vi "Prasing Frame.vi"(8 "error in (no error)":errorcluster caption="entrée d'erreur (pas d'erreur)", 11 "Class UART Enocean en entrée":refnum<class "Class UART Enocean.lvclass">) -> (0 "error out":errorcluster caption="sortie d'erreur", 3 "Class UART Enocean en sortie":refnum<class "Class UART Enocean.lvclass">)   [LabVIEW 2020, in "Library Instrument & Equipement.lvlib" / "Library UART.lvlib" / "Class UART Enocean.lvclass"]
uses:
  Class UART Enocean.lvclass
  C:/Users/ngarcin/OneDrive - Altyor/Standard TB/Class/UART/UART (Default)/Class UART (Default).lvclass
  Class UART Enocean.lvclass/Class UART Enocean.ctl
  Commun VI/Library Commun.lvlib
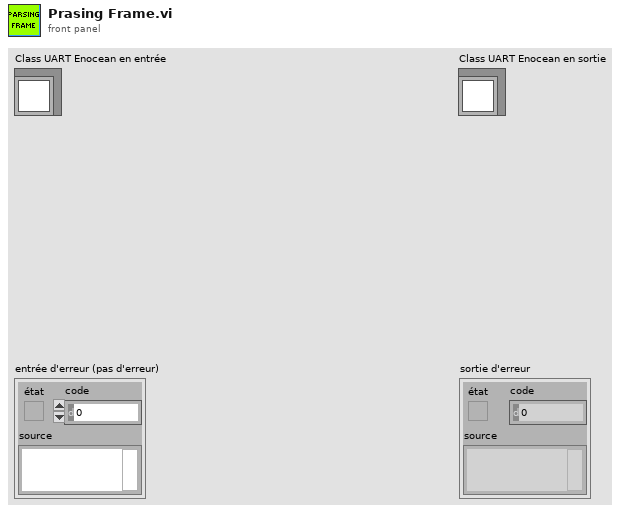
[diagram p1: front panel]
types:
  T1 = enum16{"Wait Synchro bit", "Wait Size Header", "Check CRC Header", "Wait Size Data", "Wait Size Optional", "Check CRC Data", "Extract Data"}[]
  T2 = enum16{"CRC Altyor", "CRC Xor On all Bytes", "CRC8", "CRC16", "CRC32", "Other"}
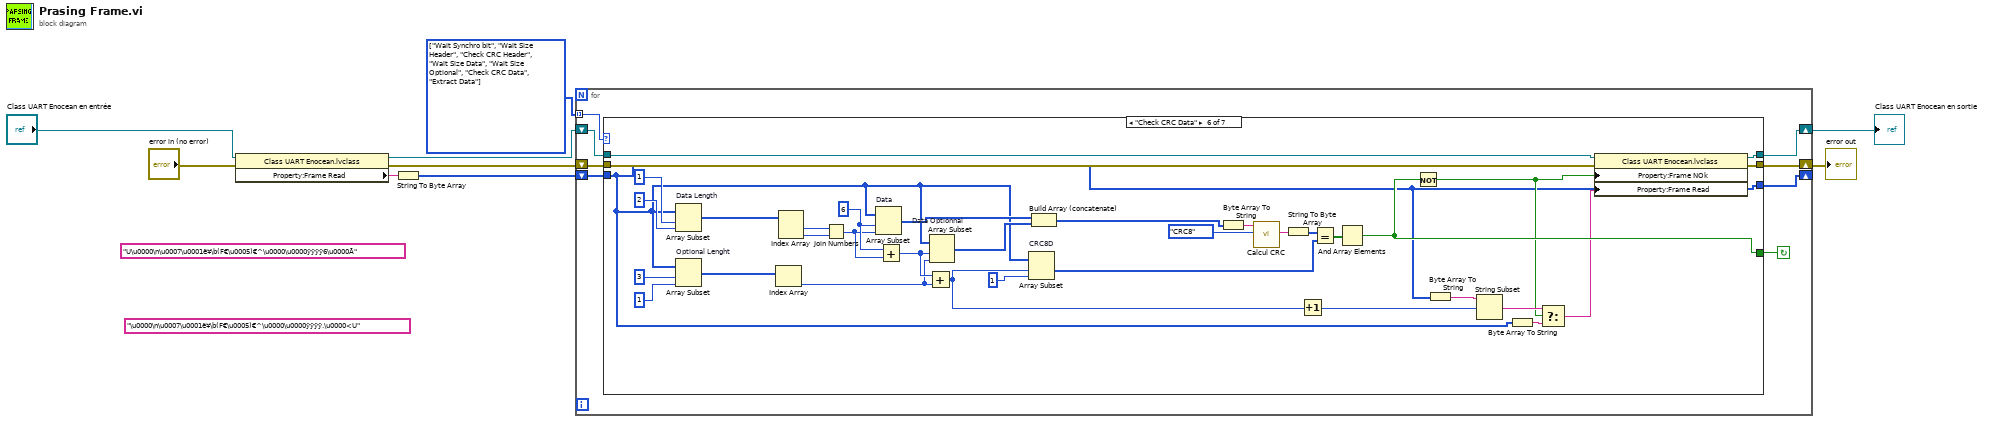
[diagram p0: block diagram]
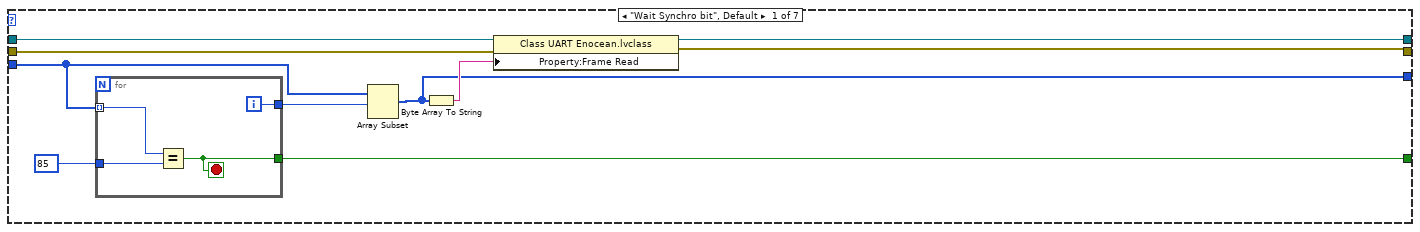
[diagram p2: hidden frame]
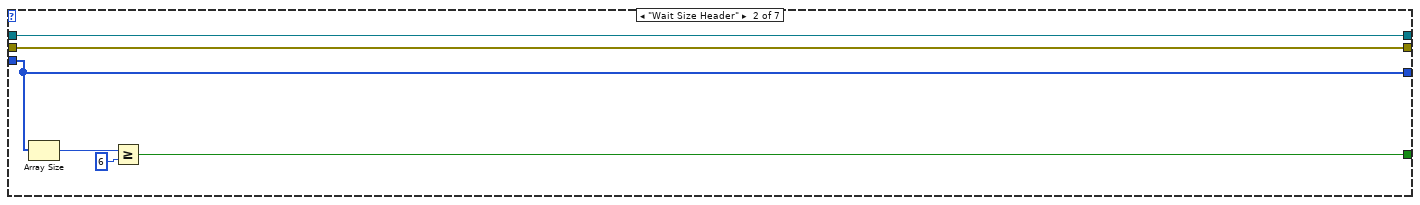
[diagram p3: hidden frame]
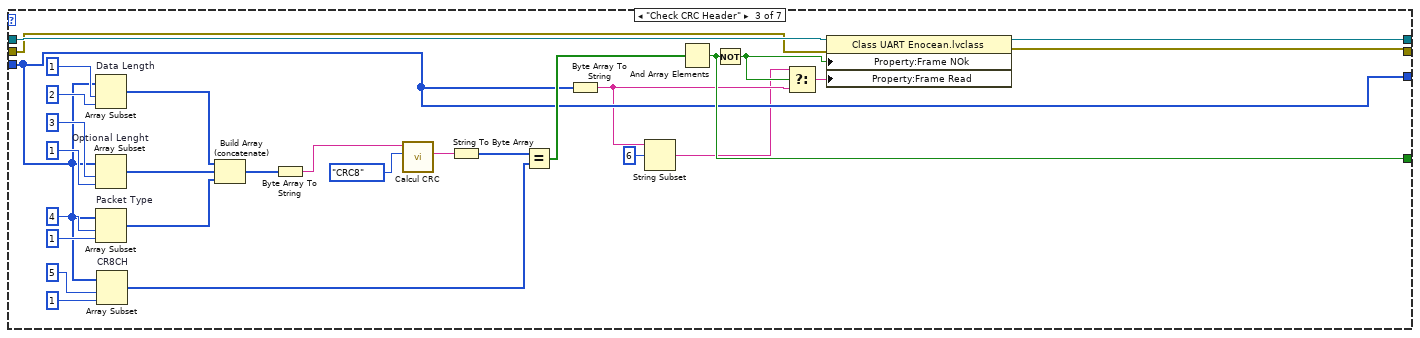
[diagram p4: hidden frame]
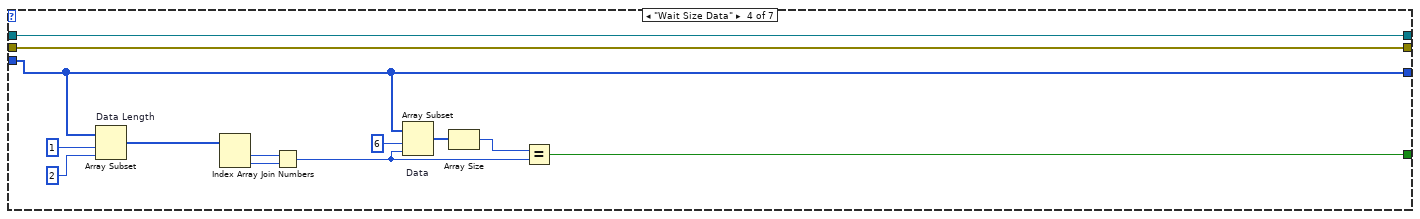
[diagram p5: hidden frame]
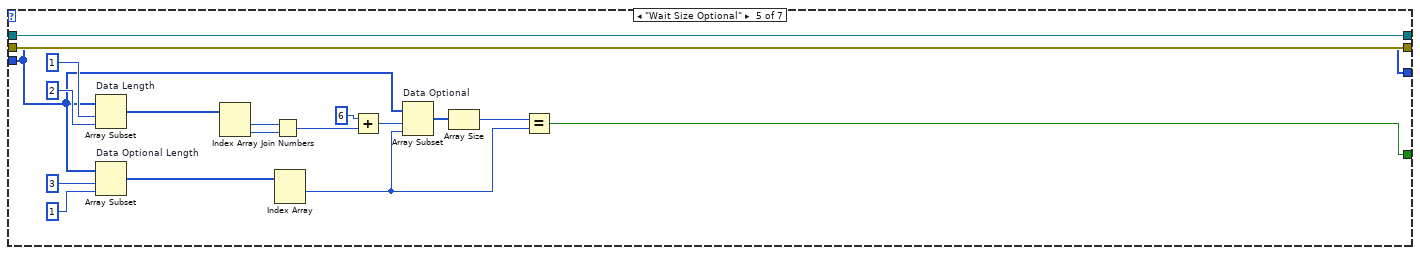
[diagram p6: hidden frame]
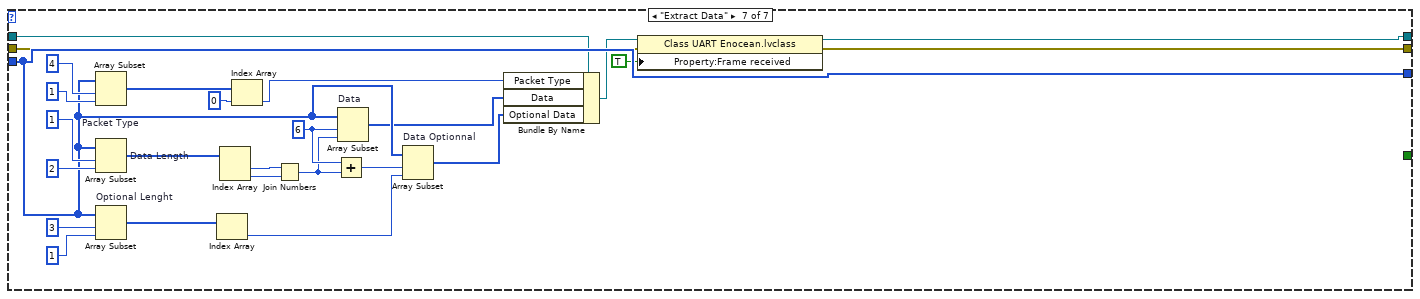
[diagram p7: hidden frame]
diagram:
  (unwired) "\u0000\n\u0007\u0001ë¥\b(F€\u0005)€^\u0000\u0000ÿÿÿÿ.\u0000<U" ("chaîne")
  (unwired) "U\u0000\n\u0007\u0001ë¥\b(F€\u0005)€^\u0000\u0000ÿÿÿÿ6\u0000Ã" ("chaîne")
  w7 = T1 [enum."Wait Synchro bit", enum."Wait Size Header", enum."Check CRC Header", enum."Wait Size Data", enum."Wait Size Optional", enum."Check CRC Data", enum."Extract Data"] items=["Wait Synchro bit", "Wait Size Header", "Check CRC Header", "Wait Size Data", "Wait Size Optional", "Check CRC Data", "Extract Data"]
  n1 = property class="Class UART Enocean.lvclass"(reference="Class UART Enocean en entrée", error in="error in (no error)") -> (reference out=w5:refnum<class "Class UART Enocean.lvclass">, error out=w2:errorcluster, "Property:Frame Read"=w1:string)
  n2 = String To Byte Array(string=w1) -> (unsigned byte array=w6:u8[])
  n3 = for {
    tunnel: w7 -> [w16] mode=indexing
    shift-right: [w13] -> w4
    shift-left: w5 -> [w14]
    shift-right: [w11] -> w3
    shift-left: w2 -> [w12]
    shift-right: [w10] -> _
    shift-left: w6 -> [w17]
    stop <- w15 continue-if-true
    n4 = case shown="\"Check CRC Data\"" w16 {
      tunnel: w17 -> [w21 w37 w43 w73 w83 w101 w144]
      tunnel: [w26 w34 w47 w70 w92 w106 _] -> w15
      tunnel: w14 -> [w25 w33 w48 w68 w91 w110 w143]
      tunnel: [w24 w33 w44 w68 w91 w109 w136] -> w13
      tunnel: w12 -> [w23 w32 w46 w67 w90 w108 w135]
      tunnel: [w22 w32 w45 w67 w90 w107 w134] -> w11
      tunnel: [w18 w37 w43 w73 w83 w101 w144] -> w10
      frame "Wait Synchro bit", Default {
        n5 = for {
          tunnel: w21 -> [w31] mode=indexing
          tunnel: [w30] -> w20
          tunnel: u8 85 -> [w29]
          tunnel: [w28] -> w26
          i -> [w30]
          stop <- w28 stop-if-true
          n6 = Equal?(x=w31, y=w29) -> (x = y?=w28:bool)
        }
        n7 = Array Subset(array=w21, index=w20) -> (w18:u8[])  [unwired: 1 in]
        n8 = Byte Array To String(unsigned byte array=w18) -> (string=w19:string)
        n9 = property class="Class UART Enocean.lvclass"(reference=w25, error in=w23, "Property:Frame Read"=w19) -> (reference out=w24:refnum<class "Class UART Enocean.lvclass">, error out=w22:errorcluster)
      }
      frame "Wait Size Header" {
        n10 = Array Size(array=w37) -> (size(s)=w36:i32)
        n11 = Greater Or Equal?(x=w36, y=6) -> (x >= y?=w34:bool)
      }
      frame "Check CRC Header" {
        n12 = Array Subset "Data Length"(array=w43, index=1 ("indice"), length=2 ("longueur")) -> (w55:u8[])
        n13 = Array Subset "Optional Lenght"(array=w43, index=3 ("indice"), length=1 ("longueur")) -> (w63:u8[])
        n14 = Array Subset "Packet Type"(array=w43, index=4 ("indice"), length=1 ("longueur")) -> (w62:u8[])
        n15 = Array Subset "CR8CH"(array=w43, index=5 ("indice"), length=1 ("longueur")) -> (w57:u8[])
        n16 = Build Array (concatenate)(w55, w63, w62) -> (w61:u8[])
        n17 = Byte Array To String(unsigned byte array=w61) -> (string=w60:string)
        n18 = call "Calcul CRC.vi"("CRC type"=T2."CRC8", "Trame"=w60) -> ("CRC"=w59:string)  [unwired: 8 in, 1 out]
        n19 = String To Byte Array(string=w59) -> (unsigned byte array=w58:u8[])
        n20 = Equal?(x=w58, y=w57) -> (x = y?=w56:bool[])
        n21 = Byte Array To String(unsigned byte array=w43) -> (string=w40:string)
        n22 = String Subset(string=w40, offset (0)=6) -> (substring=w38:string)  [unwired: 1 in]
        n23 = And Array Elements(Boolean array=w56) -> (logical AND=w47:bool)
        n24 = Not(x=w47) -> (.not. x?=w42:bool)
        n25 = Select(t=w38, s=w42, f=w40) -> (s? t:f=w41:string)
        n26 = property class="Class UART Enocean.lvclass"(reference=w48, error in=w46, "Property:Frame NOk"=w42, "Property:Frame Read"=w41) -> (reference out=w44:refnum<class "Class UART Enocean.lvclass">, error out=w45:errorcluster)
      }
      frame "Wait Size Data" {
        n27 = Array Subset "Data Length"(array=w73, index=1 ("indice"), length=2 ("longueur")) -> (w78:u8[])
        n28 = Index Array(array=w78) -> (element #1=w77:u8, element #2=w76:u8)  [unwired: 2 in]
        n29 = Join Numbers(hi=w77, lo=w76) -> ((hi.lo)=w69:u16)
        n30 = Array Subset "Data"(array=w73, index=6 ("indice"), length=w69) -> (w75:u8[])
        n31 = Array Size(array=w75) -> (size(s)=w74:i32)
        n32 = Equal?(x=w74, y=w69) -> (x = y?=w70:bool)
      }
      frame "Wait Size Optional" {
        n33 = Array Subset "Data Length"(array=w83, index=1 ("indice"), length=2 ("longueur")) -> (w88:u8[])
        n34 = Array Subset "Data Optional Length"(array=w83, index=3 ("indice"), length=1 ("longueur")) -> (w97:u8[])
        n35 = Index Array(array=w88) -> (element #1=w87:u8, element #2=w86:u8)  [unwired: 2 in]
        n36 = Join Numbers(hi=w87, lo=w86) -> ((hi.lo)=w82:u16)
        n37 = Index Array(array=w97) -> (element #1=w89:u8)  [unwired: 2 in, 1 out]
        n38 = Add(x=6 ("indice"), y=w82) -> (x+y=w80:i32)
        n39 = Array Subset "Data Optional"(array=w83, index=w80, length=w89) -> (w96:u8[])
        n40 = Array Size(array=w96) -> (size(s)=w95:i32)
        n41 = Equal?(x=w95, y=w89) -> (x = y?=w92:bool)
      }
      frame "Check CRC Data" {
        w119 = 6 ("indice")
        n42 = Array Subset "Data Length"(array=w101, index=1 ("indice"), length=2 ("longueur")) -> (w132:u8[])
        n43 = Array Subset "Optional Lenght"(array=w101, index=3 ("indice"), length=1 ("longueur")) -> (w117:u8[])
        n44 = Index Array(array=w117) -> (element=w113:u8)  [unwired: 1 in]
        n45 = Index Array(array=w132) -> (element #1=w131:u8, element #2=w130:u8)  [unwired: 2 in]
        n46 = Join Numbers(hi=w131, lo=w130) -> ((hi.lo)=w118:u16)
        n47 = Array Subset "Data"(array=w101, index=w119, length=w118) -> (w120:u8[])
        n48 = Add(x=w119, y=w118) -> (x+y=w114:i32)
        n49 = Add(x=w114, y=w113) -> (x+y=w99:i32)
        n50 = Array Subset "Data Optionnal"(array=w101, index=w114, length=w113) -> (w112:u8[])
        n51 = Array Subset "CRC8D"(array=w101, index=w99, length=1 ("longueur")) -> (w111:u8[])
        n52 = Build Array (concatenate)(w120, w112) -> (w122:u8[])
        n53 = Byte Array To String(unsigned byte array=w122) -> (string=w123:string)
        n54 = call "Calcul CRC.vi"("CRC type"=T2."CRC8", "Trame"=w123) -> ("CRC"=w124:string)  [unwired: 8 in, 1 out]
        n55 = String To Byte Array(string=w124) -> (unsigned byte array=w125:u8[])
        n56 = Increment(x=w99) -> (x+1=w98:i32)
        n57 = Equal?(x=w125, y=w111) -> (x = y?=w116:bool[])
        n58 = And Array Elements(Boolean array=w116) -> (logical AND=w106:bool)
        n59 = Not(x=w106) -> (.not. x?=w102:bool)
        n60 = Byte Array To String(unsigned byte array=w101) -> (string=w100:string)
        n61 = String Subset(string=w100, offset (0)=w98) -> (substring=w105:string)  [unwired: 1 in]
        n62 = Byte Array To String(unsigned byte array=w101) -> (string=w104:string)
        n63 = Select(t=w105, s=w102, f=w104) -> (s? t:f=w103:string)
        n64 = property class="Class UART Enocean.lvclass"(reference=w110, error in=w108, "Property:Frame NOk"=w102, "Property:Frame Read"=w103) -> (reference out=w109:refnum<class "Class UART Enocean.lvclass">, error out=w107:errorcluster)
      }
      frame "Extract Data" {
        w151 = 6 ("indice")
        n65 = Array Subset "Packet Type"(array=w144, index=4 ("indice"), length=1 ("longueur")) -> (w142:u8[])
        n66 = Array Subset "Data Length"(array=w144, index=1 ("indice"), length=2 ("longueur")) -> (w158:u8[])
        n67 = Array Subset "Optional Lenght"(array=w144, index=3 ("indice"), length=1 ("longueur")) -> (w149:u8[])
        n68 = Index Array(array=w149) -> (element=w147:u8)  [unwired: 1 in]
        n69 = Index Array(array=w158) -> (element #1=w157:u8, element #2=w156:u8)  [unwired: 2 in]
        n70 = Index Array(array=w142, index=0 ("indice")) -> (element=w141:u8)
        n71 = Join Numbers(hi=w157, lo=w156) -> ((hi.lo)=w150:u16)
        n72 = Add(x=w151, y=w150) -> (x+y=w148:i32)
        n73 = Array Subset "Data"(array=w144, index=w151, length=w150) -> (w140:u8[])
        n74 = Array Subset "Data Optionnal"(array=w144, index=w148, length=w147) -> (w139:u8[])
        n75 = Bundle By Name(cluster=w143, "Packet Type"=w141, "Data"=w140, "Optional Data"=w139) -> (w138:refnum<class "Class UART Enocean.lvclass">)
        n76 = property class="Class UART Enocean.lvclass"(reference=w138, error in=w135, "Property:Frame received"=TRUE ("Frame received")) -> (reference out=w136:refnum<class "Class UART Enocean.lvclass">, error out=w134:errorcluster)
      }
    }
  }
  "error out" <- w3
  "Class UART Enocean en sortie" <- w4
